vi "Send FPGA Telemetry.vi"   [LabVIEW 2015]
uses:
  Session Information.ctl
  FPGA Telemetry.ctl
  Vehicle Status/Subsystem Status.ctl
  Vehicle Status/Subsystem Status Severity.ctl
  Vehicle Status/Subsystem Status Message.ctl
  AIR Status.ctl
  Reason for Shutdown.ctl
  Dash LED Status.ctl
  FPGA/SPI v2/ADXL345 Output.ctl
  Global Data.vi
  <vilib>/FPGAPlugInAG/sbRIO-9627/niLvFpga_Open_sbRIO-9627.vi
  <vilib>/rvi/interface/common/dynamic/niFpgaDynamicAddResources.vi
  <vilib>/Utility/error.llb/Error Cluster From Error Code.vi
  <vilib>/rvi/errors/niLvFpgaAdjustHostInterfaceError.vi
  <vilib>/FPGAPlugInAG/Dynamic/niLvFpga_Close_Dynamic.vi
  <vilib>/rvi/interface/nirviOpenFPGA/nirviOpenFPGA.xnode
  FPGA Bitfiles/Latest.lvbitx
  <vilib>/rvi/interface/nirviReadWriteControl/nirviReadWriteControl.xnode
  <vilib>/rvi/interface/nirviCloseFPGA/nirviCloseFPGA.xnode
  <vilib>/NI_Real-Time Target Support.lvlib
  NiFpgaLv.dll
  <vilib>/rvi/interface/Simulation/niFpgaSimulationCallBeginRW.vi
types:
  T1 = typedef "Session Information.ctl" = cluster{"CLogFilePrefix":string, "CExtraNotes":string, "CCircuit":string, "CCarName":string, "CDriverName":string, "CSessionDescription":string}
  T2 = typedef "FPGA Telemetry.ctl" = cluster{"CPU Load":cluster{"Total (%)":dbl, "Time Critical (%)":dbl, "Timed Structures (%)":dbl, "High (%)":dbl, "Above Normal (%)":dbl, "Normal (%)":dbl, "Background (%)":dbl, "Idle (%)":dbl, "ISR (%)":dbl}, "SVehicleStatus":cluster{"BMS Status":T3, "MC Status":T3, "Shutdown Status":T3, "sbRIO Status":T3, "Vehicle Status":T3, "Shutdown State":enum16{"NI.SC.Initial", "NI.SC.History", "NI.SC.ShallowHistory", "NI.SC.Terminal", "Coolant Pump Started/AIR's On", "AIRs On", "Precharge", "TSMS Off"}, "AIR Status":T6, "Remote Return to Pits":bool, "Reason for Shutdown":T7, "MC State Machine Status":enum16{"NI.SC.Initial", "NI.SC.History", "NI.SC.ShallowHistory", "NI.SC.Terminal", "Broadcast Diag", "Let Current Drop then Disable AIR's", "Enabled", "Disabled"}}, "iPhone HF Data":cluster{"gXiPhone":dbl, "gYiPhone":dbl, "gZiPhone":dbl, "nYawXiPhone":dbl, "nYawYiPhone":dbl, "nYawZiPhone":dbl}, "iPhone LF Data":cluster{"nLatiPhone":dbl, "nLongiPhone":dbl, "nGPSiPhone":dbl}, "stop":bool, "VSupplyOffset":fxp<+,12,4>, "VsbRIOSupply":fxp<+/-,25,6>, "bFPGALED":bool, "TSBRIO":fxp<+/-,33,17>, "rTPS2Unscaled":fxp<+/-,16,1>, "rTPS1Unscaled":fxp<+/-,16,1>, "bTPSConsistent":bool, "bTPSInRange":bool, "rThrottle":fxp<+/-,33,22>, "VTPS2":fxp<+/-,24,5>, "rTPS2":fxp<+/-,31,22>, "VTPS1":fxp<+/-,24,5>, "rTPS1":fxp<+/-,31,22>, "rTPS2Max":fxp<+,16,4>, "rTPS2Min":fxp<+,16,4>, "rTPS1Max":fxp<+,16,4>, "rTPS1Min":fxp<+,16,4>, "bCoolantPumpEnable":bool, "bRTDSEnable":bool, "bTSMSInStatus":bool, "bPosAIREnable":bool, "bBMSOK":bool, "bIMDOK":bool, "bBSPDOK":bool, "bSBRIOOK2":bool, "bSBRIOOK1":bool, "bTSMSOutStatus":bool, "eGreenDash":T8, "eYellowDash":T8, "eRedDash":T8, "bMotorControllerEnable":bool, "tCurrentLap":u32, "bNewLap":bool, "tLastLap":u32, "tLapMin":u32, "V5VSupply":fxp<+/-,24,5>, "bWheelRL":bool, "bWheelRR":bool, "bWheelFR":bool, "bWheelFL":bool, "VBrakePressureR":fxp<+/-,24,5>, "VBrakePressureF":fxp<+/-,24,5>, "bWheelRRStopped":bool, "bWheelRLStopped":bool, "bWheelFRStopped":bool, "bWheelFLStopped":bool, "tWheelRLPeriod":u32, "tWheelRRPeriod":u32, "tWheelFRPeriod":u32, "tWheelFLPeriod":u32, "bBrakeLight":bool, "VShockRR":fxp<+/-,24,5>, "VShockRL":fxp<+/-,24,5>, "VShockFR":fxp<+/-,24,5>, "VShockFL":fxp<+/-,24,5>, "IHighCurrent":fxp<+/-,24,15>, "ILowCurrent":fxp<+/-,24,15>, "pBrakeR":fxp<+,26,13>, "pBrakeF":fxp<+,26,13>, "bHighCurrentOK":bool, "bLowCurrentOK":bool, "bBrakeROK":bool, "bBrakeFOK":bool, "VSteerWheelMiddle":fxp<+/-,26,5>, "aSteerWheel":fxp<+/-,31,13>, "nWheelFL":fxp<+/-,32,16>, "nWheelFR":fxp<+/-,32,16>, "nWheelRL":fxp<+/-,32,16>, "nWheelRR":fxp<+/-,32,16>, "ADXL345 Output":T9, "Tire Diameter(m)":fxp<+,16,1>, "vWheelRR":fxp<+/-,32,18>, "vWheelRL":fxp<+/-,32,18>, "vWheelFR":fxp<+/-,32,18>, "vWheelFL":fxp<+/-,32,18>, "vWheelLowest":fxp<+/-,32,18>, "vWheelHighest":fxp<+/-,32,18>, "bAccel":bool, "vAxleF":fxp<+/-,33,19>, "vCar":fxp<+/-,33,19>, "sLap":fxp<+,32,12>, "rSlipRL":fxp<+/-,12,1>, "rSlipRR":fxp<+/-,12,1>, "rSlipFL":fxp<+/-,12,1>, "rSlipFR":fxp<+/-,12,1>, "NLap":u8, "tLapReference":u32, "tFastestLap":u32, "MTorqueRequest":dbl, "RS232 Error Out":cluster{"status":bool, "code":i32}}
  T3 = typedef "Subsystem Status.ctl" = cluster{"eStatusSeverity":T4, "NValue":sgl, "CMessage":T5, "bNotOK":bool}
  T4 = typedef "Subsystem Status Severity.ctl" = enum16{"Okay", "Short Warning", "Long Warning", "Return to Pits", "Error", "Danger"}
  T5 = typedef "Subsystem Status Message.ctl" = enum16{"ControllerTemperature", "MotorTemperature", "BatteryTemperature", "BatteryLowVoltage", "LVBattery", "sbRIOTemperature", "Precharge", "BSPD", "IMD", "RemoteReturnToPits", "EStopInterrupted", "NoCellComms", "MCOverSpeed", "MCOverCurrent", "MCOverVoltage", "MCInverterOverTemp", "MCDirectionCommand", "MCInverterTimeout", "MCDesatFault", "MCHWOverCurrent", "MCUnderVoltage", "MCCommandMessageLost", "MotorOverTemp", "MCModAOverTemp", "MCModBOverTemp", "MCModCOverTemp", "MCPCBOverTemp", "MCGateDrv1OverTemp", "MCDateDrv2OverTemp", "MCCurrentSensorFault", "MCResolverNotConnected", "ShutdownLatchTripped", "UnknownBMS", "RemoteEmergency"}
  T6 = typedef "AIR Status.ctl" = enum16{"Off", "Precharge", "On"}
  T7 = typedef "Reason for Shutdown.ctl" = enum16{"None", "BMS", "Shutdown", "sbRIO", "MC", "Remote"}
  T8 = typedef "Dash LED Status.ctl" = enum16{"Off", "Flashing", "On"}
  T9 = typedef "ADXL345 Output.ctl" = cluster{"X":fxp<+/-,14,4>, "Y":fxp<+/-,14,4>, "Z":fxp<+/-,14,4>}
  T10 = typedef "NI_Real-Time Target Support.lvlib/RT CPU Load.ctl" = cluster{"Total (%)":dbl, "Time Critical (%)":dbl, "Timed Structures (%)":dbl, "High (%)":dbl, "Above Normal (%)":dbl, "Normal (%)":dbl, "Background (%)":dbl, "Idle (%)":dbl, "ISR (%)":dbl}
  T11 = typedef "Shutdown State Machine.lvsc/State.ctl" = enum16{"NI.SC.Initial", "NI.SC.History", "NI.SC.ShallowHistory", "NI.SC.Terminal", "Coolant Pump Started/AIR's On", "AIRs On", "Precharge", "TSMS Off"}
  T12 = cluster{"X":fxp<+/-,14,4>, "Y":fxp<+/-,14,4>, "Z":fxp<+/-,14,4>}
  T13 = typedef "MC State Machine.lvsc/State.ctl" = enum16{"NI.SC.Initial", "NI.SC.History", "NI.SC.ShallowHistory", "NI.SC.Terminal", "Broadcast Diag", "Let Current Drop then Disable AIR's", "Enabled", "Disabled"}
  T14 = cluster{"Accel X":dbl, "Accel Y":dbl, "Accel Z":dbl, "Gyro X":dbl, "Gyro Y":dbl, "Gyro Z":dbl}
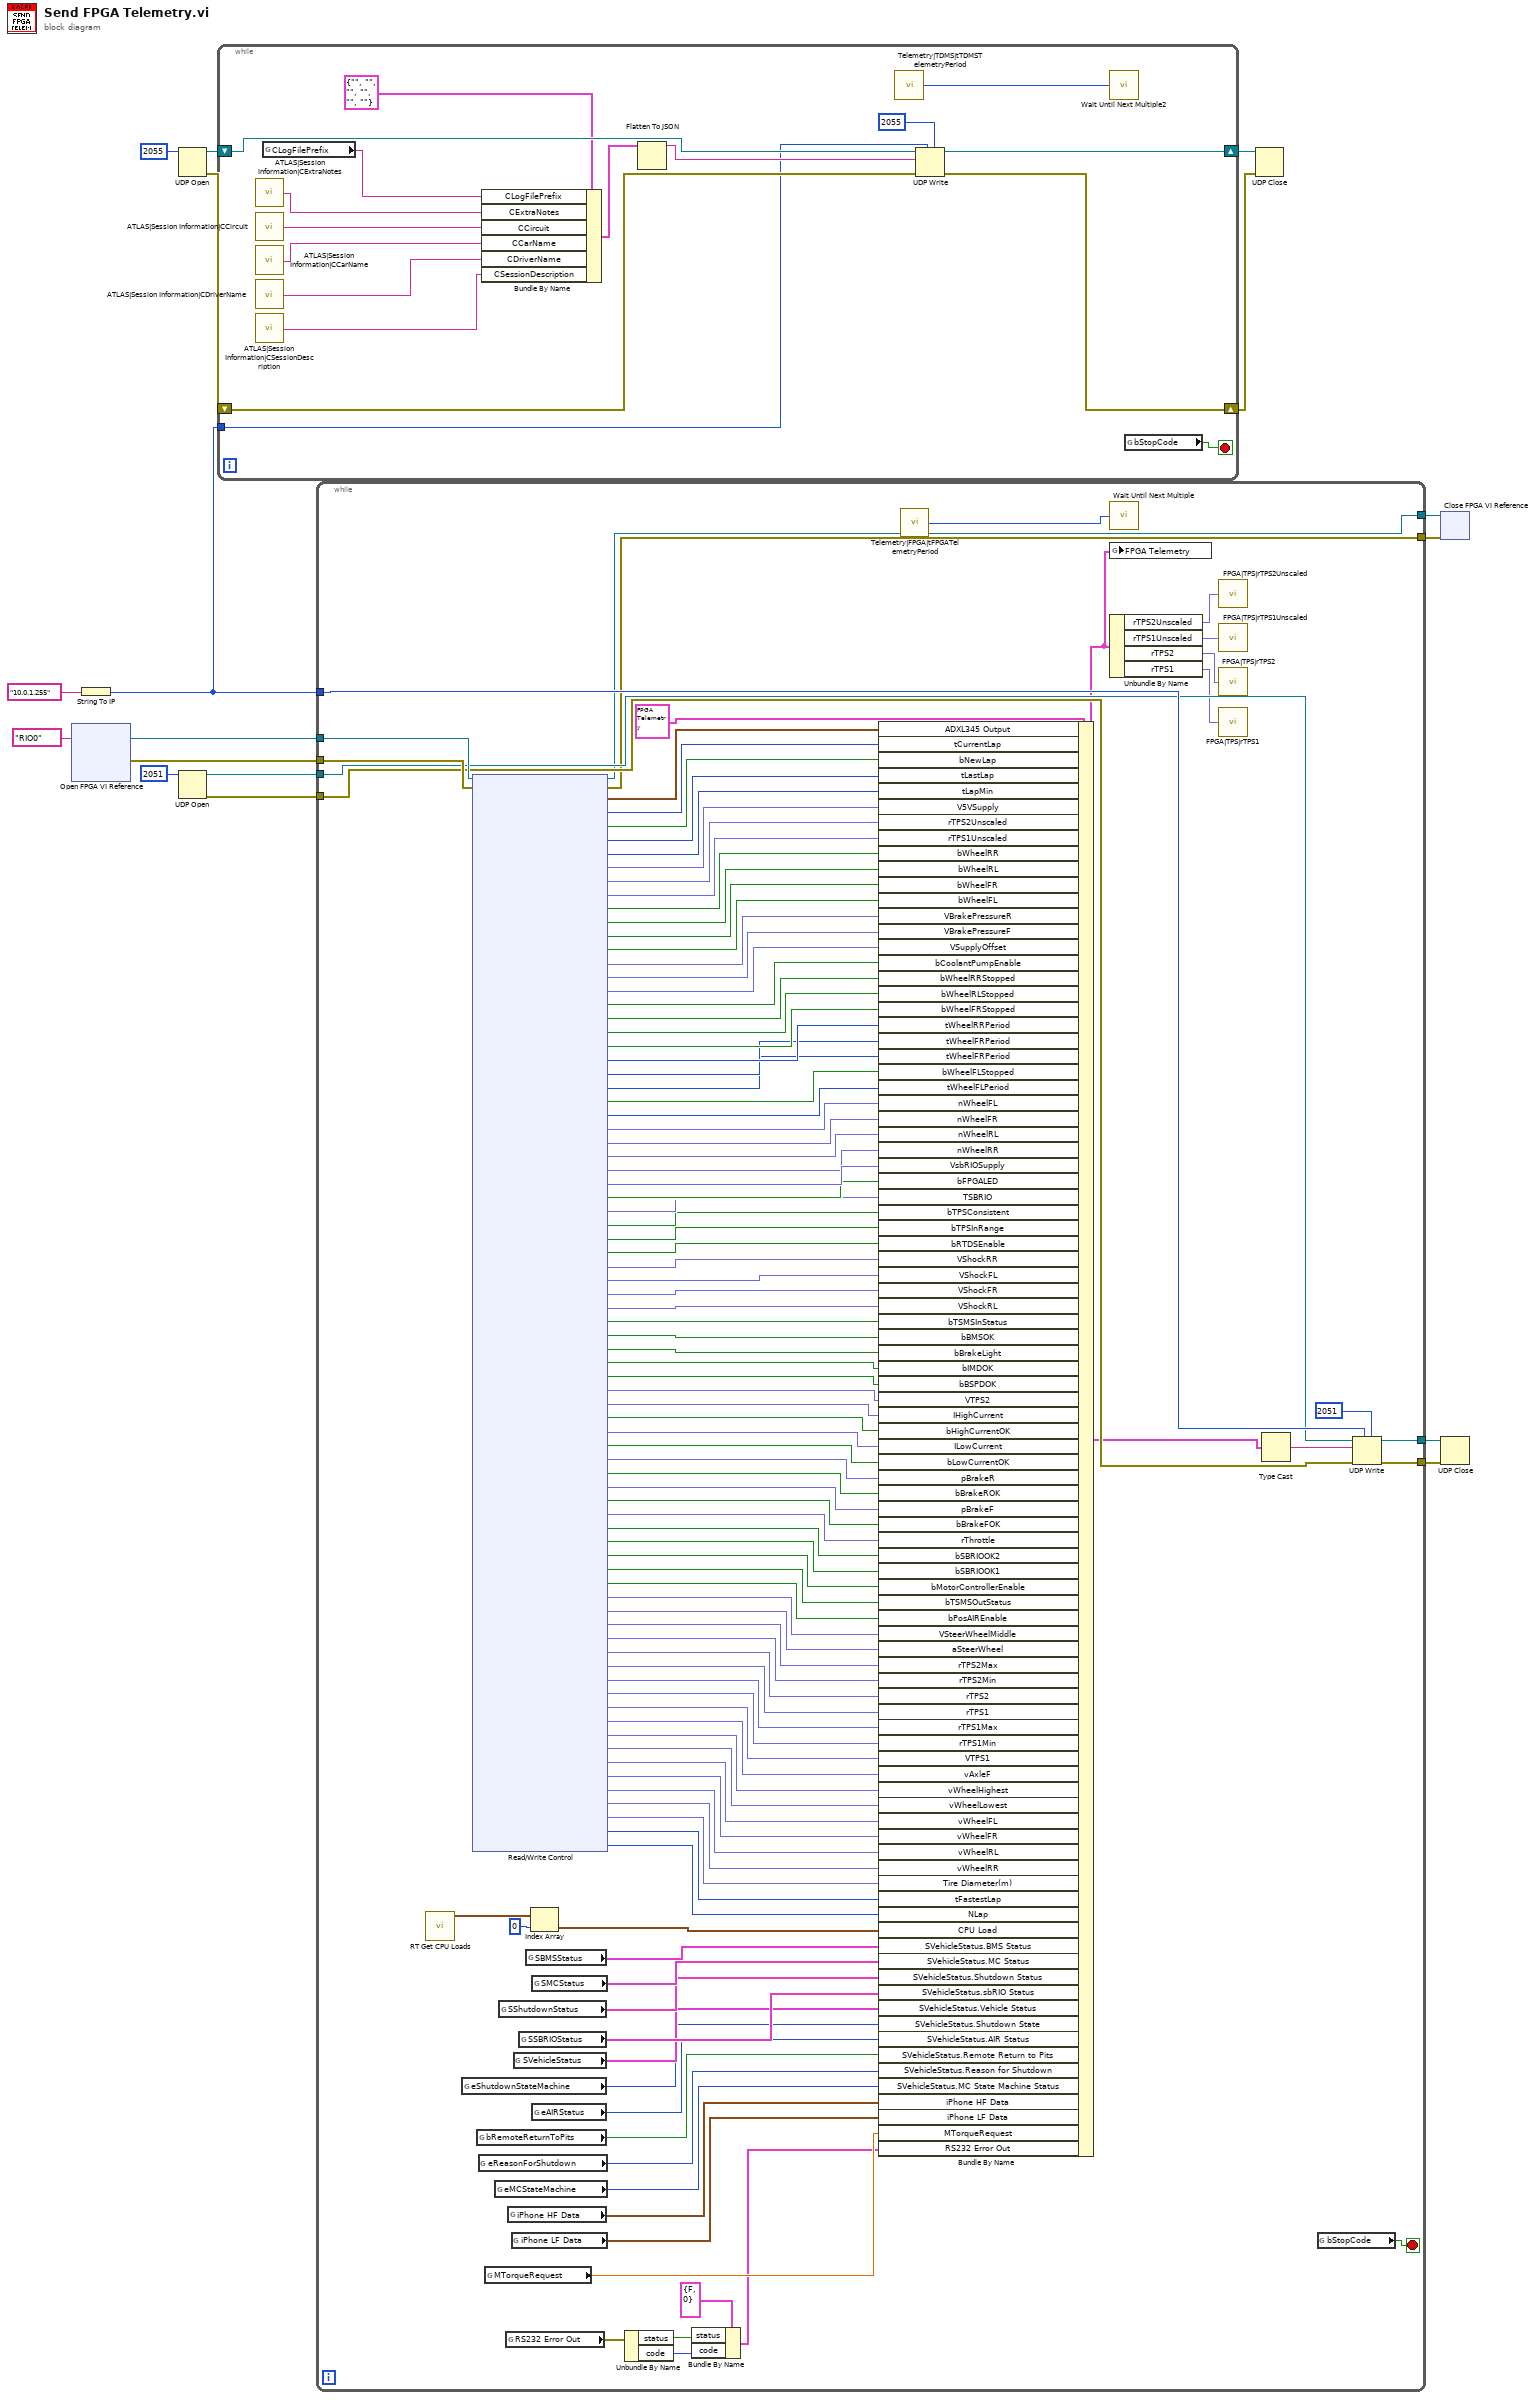
[diagram p0: block diagram]
diagram:
  n1 = xnode "Open FPGA VI Reference"("resource name"=tag "RIO0") -> ("FPGA VI Reference Out"=w17:refnum<k20>, "error out"=w16:errorcluster)  [unwired: 1 in]
  n2 = String To IP(1:"10.0.1.255" ("net address")) -> (0:w5:u32)
  n3 = UDP Open(11:u16 2055 ("port")) -> (port=w7:refnum<k16>, 0:w6:errorcluster)  [unwired: 4 in, 1 out]
  n4 = UDP Open(11:u16 2051 ("port")) -> (port=w10:refnum<k16>, 0:w9:errorcluster)  [unwired: 4 in, 1 out]
  n5 = while {
    tunnel: w5 -> [w30]
    shift-right: [w29] -> w2
    shift-left: w7 -> [w33]
    shift-right: [w28] -> w3
    shift-left: w6 -> [w32]
    stop <- w27 stop-if-true
    n6 = call "ATLAS|Session Information|CExtraNotes"() -> ("Value"=w22:string)
    n7 = call "ATLAS|Session Information|CCircuit"() -> ("Value"=w21:string)
    n8 = call "ATLAS|Session Information|CCarName"() -> ("Value"=w20:string)
    n9 = call "ATLAS|Session Information|CDriverName"() -> ("Value"=w19:string)
    n10 = call "ATLAS|Session Information|CSessionDescription"() -> ("Value"=w18:string)
    n11 = global read "Global Data.vi" "CLogFilePrefix"() -> (w24:string)
    n12 = Bundle By Name(cluster=T1 {"CLogFilePrefix"="", "CExtraNotes"="", "CCircuit"="", "CCarName"="", "CDriverName"="", "CSessionDescription"=""} ("Session Information"), "CLogFilePrefix"=w24, "CExtraNotes"=w22, "CCircuit"=w21, "CCarName"=w20, "CDriverName"=w19, "CSessionDescription"=w18) -> (w23:T1)
    n13 = Flatten To JSON(anything=w23) -> (JSON string=w34:string)  [unwired: 2 in, 1 out]
    n14 = call "Telemetry|TDMS|tTDMSTelemetryPeriod"() -> ("Value"=w26:u32)
    n15 = UDP Write(address=w30, port or service name=u16 2055, connection ID=w33, data in=w34, 8:w32) -> (error out=w28:errorcluster, 3:w29:refnum<k16>)  [unwired: 1 in]
    n16 = call "Wait Until Next Multiple2"("Count(mSec)"=w26) -> ()  [unwired: 1 out]
    n17 = global read "Global Data.vi" "bStopCode"() -> (w27:bool)
  }
  n18 = while {
    tunnel: w17 -> [w151]
    tunnel: w16 -> [w150]
    tunnel: w5 -> [w148]
    tunnel: w10 -> [w146]
    tunnel: w9 -> [w145]
    tunnel: [w144] -> w14
    tunnel: [w143] -> w13
    tunnel: [w142] -> w12
    tunnel: [w141] -> w11
    stop <- w61 stop-if-true
    n19 = call <vilib>:"RT Get CPU Loads.vi"() -> ("CPU loads"=w139:T10[])  [unwired: 10 in, 1 out]
    n20 = global read "Global Data.vi" "eShutdownStateMachine"() -> (w68:T11)
    n21 = xnode "Read/Write Control"("FPGA VI Reference In"=w151, "error in"=w150) -> ("FPGA VI Reference Out"=w142:refnum<k20>, "error out"=w141:errorcluster, "ADXL345 Output"=w137:T12, "tCurrentLap"=w136:u32, "bNewLap"=w135:bool, "tLastLap"=w134:u32, "tLapMin"=w133:u32, "V5VSupply"=w132:fxp<+/-,24,5>, "rTPS2Unscaled"=w131:fxp<+/-,16,1>, "rTPS1Unscaled"=w130:fxp<+/-,16,1>, "bWheelRR"=w129:bool, "bWheelRL"=w128:bool, "bWheelFR"=w127:bool, "bWheelFL"=w126:bool, "VBrakePressureR"=w125:fxp<+/-,24,5>, "VBrakePressureF"=w124:fxp<+/-,24,5>, "VSupplyOffset"=w123:fxp<+,12,4>, "bCoolantPumpEnable"=w122:bool, "bWheelRRStopped"=w121:bool, "bWheelRLStopped"=w120:bool, "bWheelFRStopped"=w119:bool, "tWheelRRPeriod"=w118:u32, "tWheelRLPeriod"=w117:u32, "tWheelFRPeriod"=w116:u32, "bWheelFLStopped"=w115:bool, "tWheelFLPeriod"=w114:u32, "nWheelFL"=w60:fxp<+/-,29,16>, "nWheelFR"=w59:fxp<+/-,29,16>, "nWheelRL"=w58:fxp<+/-,29,16>, "nWheelRR"=w57:fxp<+/-,29,16>, "VsbRIOSupply"=w113:fxp<+/-,25,6>, "bFPGALED"=w112:bool, "TSBRIO"=w111:fxp<+,19,8>, "bTPSConsistent"=w110:bool, "bTPSInRange"=w109:bool, "bRTDSEnable"=w108:bool, "VShockRR"=w107:fxp<+/-,24,5>, "VShockFL"=w106:fxp<+/-,24,5>, "VShockFR"=w105:fxp<+/-,24,5>, "VShockRL"=w104:fxp<+/-,24,5>, "bTSMSInStatus"=w103:bool, "bBMSOK"=w102:bool, "bBrakeLight"=w101:bool, "bIMDOK"=w100:bool, "bBSPDOK"=w99:bool, "VTPS2"=w98:fxp<+/-,36,9>, "IHighCurrent"=w97:fxp<+/-,19,15>, "bHighCurrentOK"=w96:bool, "ILowCurrent"=w95:fxp<+/-,19,15>, "bLowCurrentOK"=w94:bool, "pBrakeR"=w93:fxp<+,26,13>, "bBrakeROK"=w92:bool, "pBrakeF"=w91:fxp<+,26,13>, "bBrakeFOK"=w90:bool, "rThrottle"=w89:fxp<+/-,33,22>, "bSBRIOOK2"=w88:bool, "bSBRIOOK1"=w87:bool, "bMotorControllerEnable"=w86:bool, "bTSMSOutStatus"=w85:bool, "bPosAIREnable"=w84:bool, "VSteerWheelMiddle"=w83:fxp<+/-,26,5>, "aSteerWheel"=w82:fxp<+/-,22,10>, "rTPS2Max"=w81:fxp<+,16,4>, "rTPS2Min"=w80:fxp<+,16,4>, "rTPS2"=w79:fxp<+/-,31,22>, "rTPS1"=w78:fxp<+/-,31,22>, "rTPS1Max"=w77:fxp<+,16,4>, "rTPS1Min"=w76:fxp<+,16,4>, "VTPS1"=w75:fxp<+/-,36,9>, "vAxleF"=w51:fxp<+/-,33,19>, "vWheelHighest"=w50:fxp<+/-,32,18>, "vWheelLowest"=w49:fxp<+/-,32,18>, "vWheelFL"=w48:fxp<+/-,32,18>, "vWheelFR"=w47:fxp<+/-,32,18>, "vWheelRL"=w46:fxp<+/-,32,18>, "vWheelRR"=w45:fxp<+/-,32,18>, "Tire Diameter(m)"=w44:fxp<+,16,1>, "tFastestLap"=w43:u32, "NLap"=w42:u8)
    n22 = global read "Global Data.vi" "bRemoteReturnToPits"() -> (w66:bool)
    n23 = global read "Global Data.vi" "eReasonForShutdown"() -> (w65:T7)
    n24 = global read "Global Data.vi" "MTorqueRequest"() -> (w41:dbl)
    n25 = global read "Global Data.vi" "eMCStateMachine"() -> (w64:T13)
    n26 = global read "Global Data.vi" "SShutdownStatus"() -> (w71:T3)
    n27 = global read "Global Data.vi" "RS232 Error Out"() -> (w39:errorcluster)
    n28 = global read "Global Data.vi" "iPhone HF Data"() -> (w63:T14)
    n29 = global read "Global Data.vi" "iPhone LF Data"() -> (w62:cluster{"Lat":dbl, "Long":dbl, "Speed":dbl})
    n30 = global read "Global Data.vi" "SVehicleStatus"() -> (w69:T3)
    n31 = global read "Global Data.vi" "SSBRIOStatus"() -> (w70:T3)
    n32 = global read "Global Data.vi" "SBMSStatus"() -> (w73:T3)
    n33 = Index Array(array=w139, index=0) -> (element=w74:T10)
    n34 = global read "Global Data.vi" "SMCStatus"() -> (w72:T3)
    n35 = global read "Global Data.vi" "eAIRStatus"() -> (w67:T6)
    n36 = Unbundle By Name(w39) -> ("status"=w37:bool, "code"=w36:i32)
    n37 = Bundle By Name(cluster=cluster{"status":bool, "code":i32} {"status"=FALSE, "code"=0} ("RS232 Error Out"), "status"=w37, "code"=w36) -> (w35:cluster{"status":bool, "code":i32})
    n38 = Bundle By Name(cluster=T2 {"CPU Load"={"Total (%)"=0.0, "Time Critical (%)"=0.0, "Timed Structures (%)"=0.0, "High (%)"=0.0, "Above Normal (%)"=0.0, "Normal (%)"=0.0, "Background (%)"=0.0, "Idle (%)"=0.0, "ISR (%)"=0.0}, "SVehicleStatus"={"BMS Status"={"eStatusSeverity"=enum."Okay", "NValue"=0.0, "CMessage"=enum."ControllerTemperature", "bNotOK"=FALSE}, "MC Status"={"eStatusSeverity"=enum."Okay", "NValue"=0.0, "CMessage"=enum."ControllerTemperature", "bNotOK"=FALSE}, "Shutdown Status"={"eStatusSeverity"=enum."Okay", "NValue"=0.0, "CMessage"=enum."ControllerTemperature", "bNotOK"=FALSE}, "sbRIO Status"={"eStatusSeverity"=enum."Okay", "NValue"=0.0, "CMessage"=enum."ControllerTemperature", "bNotOK"=FALSE}, "Vehicle Status"={"eStatusSeverity"=enum."Short Warning", "NValue"=0.0, "CMessage"=enum."ControllerTemperature", "bNotOK"=FALSE}, "Shutdown State"=enum."NI.SC.Initial", "AIR Status"=enum."Off", "Remote Return to Pits"=FALSE, "Reason for Shutdown"=enum."BMS", "MC State Machine Status"=enum."NI.SC.Initial"}, "iPhone HF Data"={"gXiPhone"=0.0, "gYiPhone"=0.0, "gZiPhone"=0.0, "nYawXiPhone"=0.0, "nYawYiPhone"=0.0, "nYawZiPhone"=0.0}, "iPhone LF Data"={"nLatiPhone"=0.0, "nLongiPhone"=0.0, "nGPSiPhone"=0.0}, "stop"=TRUE, "VSupplyOffset"=0.0, "VsbRIOSupply"=0.0, "bFPGALED"=TRUE, "TSBRIO"=0.3482666015625, "rTPS2Unscaled"=0.0, "rTPS1Unscaled"=0.999969482421875, "bTPSConsistent"=FALSE, "bTPSInRange"=FALSE, "rThrottle"=186.34033203125, "VTPS2"=0.0, "rTPS2"=-866.732421875, "VTPS1"=1.0, "rTPS1"=2.0, "rTPS2Max"=0.27001953125, "rTPS2Min"=0.489990234375, "rTPS1Max"=0.6201171875, "rTPS1Min"=0.41015625, "bCoolantPumpEnable"=FALSE, "bRTDSEnable"=FALSE, "bTSMSInStatus"=FALSE, "bPosAIREnable"=FALSE, "bBMSOK"=FALSE, "bIMDOK"=FALSE, "bBSPDOK"=FALSE, "bSBRIOOK2"=FALSE, "bSBRIOOK1"=FALSE, "bTSMSOutStatus"=FALSE, "eGreenDash"=enum."Off", "eYellowDash"=enum."Off", "eRedDash"=enum."Off", "bMotorControllerEnable"=FALSE, "tCurrentLap"=0, "bNewLap"=FALSE, "tLastLap"=0, "tLapMin"=0, "V5VSupply"=0.0, "bWheelRL"=TRUE, "bWheelRR"=TRUE, "bWheelFR"=FALSE, "bWheelFL"=FALSE, "VBrakePressureR"=0.4820976257324219, "VBrakePressureF"=0.4808177947998047, "bWheelRRStopped"=FALSE, "bWheelRLStopped"=FALSE, "bWheelFRStopped"=FALSE, "bWheelFLStopped"=TRUE, "tWheelRLPeriod"=0, "tWheelRRPeriod"=0, "tWheelFRPeriod"=0, "tWheelFLPeriod"=0, "bBrakeLight"=TRUE, "VShockRR"=0.3793773651123047, "VShockRL"=0.3444976806640625, "VShockFR"=0.3425788879394531, "VShockFL"=0.3892974853515625, "IHighCurrent"=-20.724609375, "ILowCurrent"=4.353515625, "pBrakeR"=0.0, "pBrakeF"=0.0, "bHighCurrentOK"=FALSE, "bLowCurrentOK"=FALSE, "bBrakeROK"=FALSE, "bBrakeFOK"=FALSE, "VSteerWheelMiddle"=0.34827280044555664, "aSteerWheel"=124.90449142456055, "nWheelFL"=0.0, "nWheelFR"=0.0, "nWheelRL"=0.0, "nWheelRR"=0.0, "ADXL345 Output"={"X"=0.0, "Y"=0.0, "Z"=0.0}, "Tire Diameter(m)"=0.0, "vWheelRR"=0.0, "vWheelRL"=0.0, "vWheelFR"=0.0, "vWheelFL"=0.0, "vWheelLowest"=0.0, "vWheelHighest"=0.0, "bAccel"=FALSE, "vAxleF"=0.0, "vCar"=0.0, "sLap"=0.0, "rSlipRL"=0.0, "rSlipRR"=0.0, "rSlipFL"=0.0, "rSlipFR"=0.0, "NLap"=0, "tLapReference"=0, "tFastestLap"=0, "MTorqueRequest"=0.0, "RS232 Error Out"={"status"=FALSE, "code"=0}} ("FPGA Telemetry"), "ADXL345 Output"=w137, "tCurrentLap"=w136, "bNewLap"=w135, "tLastLap"=w134, "tLapMin"=w133, "V5VSupply"=w132, "rTPS2Unscaled"=w131, "rTPS1Unscaled"=w130, "bWheelRR"=w129, "bWheelRL"=w128, "bWheelFR"=w127, "bWheelFL"=w126, "VBrakePressureR"=w125, "VBrakePressureF"=w124, "VSupplyOffset"=w123, "bCoolantPumpEnable"=w122, "bWheelRRStopped"=w121, "bWheelRLStopped"=w120, "bWheelFRStopped"=w119, "tWheelRRPeriod"=w118, "tWheelFRPeriod"=w117, "tWheelFRPeriod"=w116, "bWheelFLStopped"=w115, "tWheelFLPeriod"=w114, "nWheelFL"=w60, "nWheelFR"=w59, "nWheelRL"=w58, "nWheelRR"=w57, "VsbRIOSupply"=w113, "bFPGALED"=w112, "TSBRIO"=w111, "bTPSConsistent"=w110, "bTPSInRange"=w109, "bRTDSEnable"=w108, "VShockRR"=w107, "VShockFL"=w106, "VShockFR"=w105, "VShockRL"=w104, "bTSMSInStatus"=w103, "bBMSOK"=w102, "bBrakeLight"=w101, "bIMDOK"=w100, "bBSPDOK"=w99, "VTPS2"=w98, "IHighCurrent"=w97, "bHighCurrentOK"=w96, "ILowCurrent"=w95, "bLowCurrentOK"=w94, "pBrakeR"=w93, "bBrakeROK"=w92, "pBrakeF"=w91, "bBrakeFOK"=w90, "rThrottle"=w89, "bSBRIOOK2"=w88, "bSBRIOOK1"=w87, "bMotorControllerEnable"=w86, "bTSMSOutStatus"=w85, "bPosAIREnable"=w84, "VSteerWheelMiddle"=w83, "aSteerWheel"=w82, "rTPS2Max"=w81, "rTPS2Min"=w80, "rTPS2"=w79, "rTPS1"=w78, "rTPS1Max"=w77, "rTPS1Min"=w76, "VTPS1"=w75, "vAxleF"=w51, "vWheelHighest"=w50, "vWheelLowest"=w49, "vWheelFL"=w48, "vWheelFR"=w47, "vWheelRL"=w46, "vWheelRR"=w45, "Tire Diameter(m)"=w44, "tFastestLap"=w43, "NLap"=w42, "CPU Load"=w74, "SVehicleStatus.BMS Status"=w73, "SVehicleStatus.MC Status"=w72, "SVehicleStatus.Shutdown Status"=w71, "SVehicleStatus.sbRIO Status"=w70, "SVehicleStatus.Vehicle Status"=w69, "SVehicleStatus.Shutdown State"=w68, "SVehicleStatus.AIR Status"=w67, "SVehicleStatus.Remote Return to Pits"=w66, "SVehicleStatus.Reason for Shutdown"=w65, "SVehicleStatus.MC State Machine Status"=w64, "iPhone HF Data"=w63, "iPhone LF Data"=w62, "MTorqueRequest"=w41, "RS232 Error Out"=w35) -> (w40:T2)
    n39 = call "Telemetry|FPGA|tFPGATelemetryPeriod"() -> ("Value"=w56:u32)
    n40 = call "Wait Until Next Multiple"("Count(mSec)"=w56) -> ()  [unwired: 1 out]
    n41 = global write "Global Data.vi" "FPGA Telemetry"(w40) -> ()
    n42 = Unbundle By Name(w40) -> ("rTPS2Unscaled"=w55:fxp<+/-,16,1>, "rTPS1Unscaled"=w54:fxp<+/-,16,1>, "rTPS2"=w53:fxp<+/-,31,22>, "rTPS1"=w52:fxp<+/-,31,22>)
    n43 = call "FPGA|TPS|rTPS2Unscaled"("Value"=w55) -> ()
    n44 = call "FPGA|TPS|rTPS1Unscaled"("Value"=w54) -> ()
    n45 = call "FPGA|TPS|rTPS2"("Value"=w53) -> ()
    n46 = call "FPGA|TPS|rTPS1"("Value"=w52) -> ()
    n47 = Type Cast(x=w40) -> (*(type *) &x=w149:string)  [unwired: 1 in]
    n48 = global read "Global Data.vi" "bStopCode"() -> (w61:bool)
    n49 = UDP Write(address=w148, port or service name=u16 2051, connection ID=w146, data in=w149, 8:w145) -> (error out=w143:errorcluster, 3:w144:refnum<k16>)  [unwired: 1 in]
  }
  n50 = UDP Close(connection ID=w2, 8:w3) -> ()  [unwired: 2 out]
  n51 = xnode "Close FPGA VI Reference"("FPGA VI Reference In"=w12, "error in"=w11) -> ()  [unwired: 1 out]
  n52 = UDP Close(connection ID=w14, 8:w13) -> ()  [unwired: 2 out]
